vi "S2DS_User Instrument Initialize VIs.vi"(3 "error in":errorcluster, 4 "Port list (in)":T1, 5 "Instrument Info (in)":T2) -> (0 "error out":errorcluster, 1 "Port lists (out)":T1, 2 "Instrument info (out)":T2)   [LabVIEW 2025]
uses:
  TYPE DEFS/S2DS_Instrument Info.ctl
  TYPE DEFS/S2DS_Instrument parameters.ctl
  TYPE DEFS/S2DS_Port lists.ctl
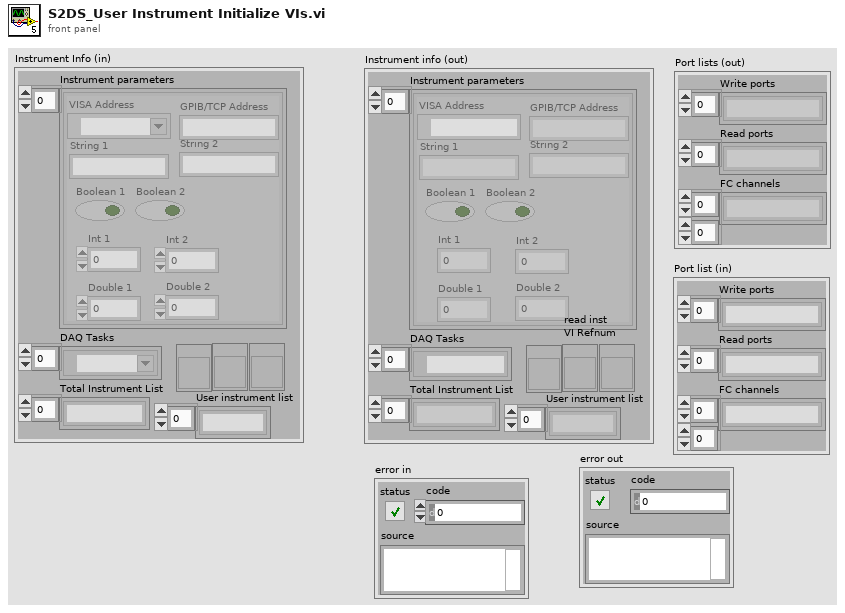
[diagram p1: front panel]
types:
  T1 = typedef "S2DS_Port lists.ctl" = cluster{"Write ports":string[], "Read ports":string[], "FC channels":string[][]}
  T2 = typedef "S2DS_Instrument Info.ctl" = cluster{"Instrument parameters":T3[], "DAQ Tasks":refnum<k21>[], "Total Instrument List":string[], "read inst \nVI Refnum":refnum<vi>, "type specifier Edit instruments VI Refnum":refnum<vi>, "type specifier write instrument VI Refnum (for type only)":refnum<vi>, "User instrument list":string[]}
  T3 = typedef "S2DS_Instrument parameters.ctl" = cluster{"VISA Address":refnum<visa-resource-name>, "GPIB/TCP Address":string, "String 1":string, "String 2":string, "Boolean 1":bool, "Boolean 2":bool, "Int 1":i32, "Int 2":i32, "Double 1":dbl, "Double 2":dbl}
  T4 = typedef "Port lists.ctl" = cluster{"Write ports":string[], "Read ports":string[], "FC channels":string[][]}
  T5 = typedef "Instrument Info.ctl" = cluster{"Instrument parameters":T6[], "DAQ Tasks":refnum<k21>[], "Instrument List":string[], "read inst \nVI Refnum":refnum<vi>, "type specifier Edit instruments VI Refnum":refnum<vi>, "type specifier write instrument VI Refnum (for type only)":refnum<vi>, "Available instrument list":string[]}
  T6 = typedef "Instrument parameters.ctl" = cluster{"VISA Address":refnum<visa-resource-name>, "GPIB/TCP Address":string, "String 1":string, "String 2":string, "Boolean 1":bool, "Boolean 2":bool, "Int 1":i32, "Int 2":i32, "Double 1":dbl, "Double 2":dbl}
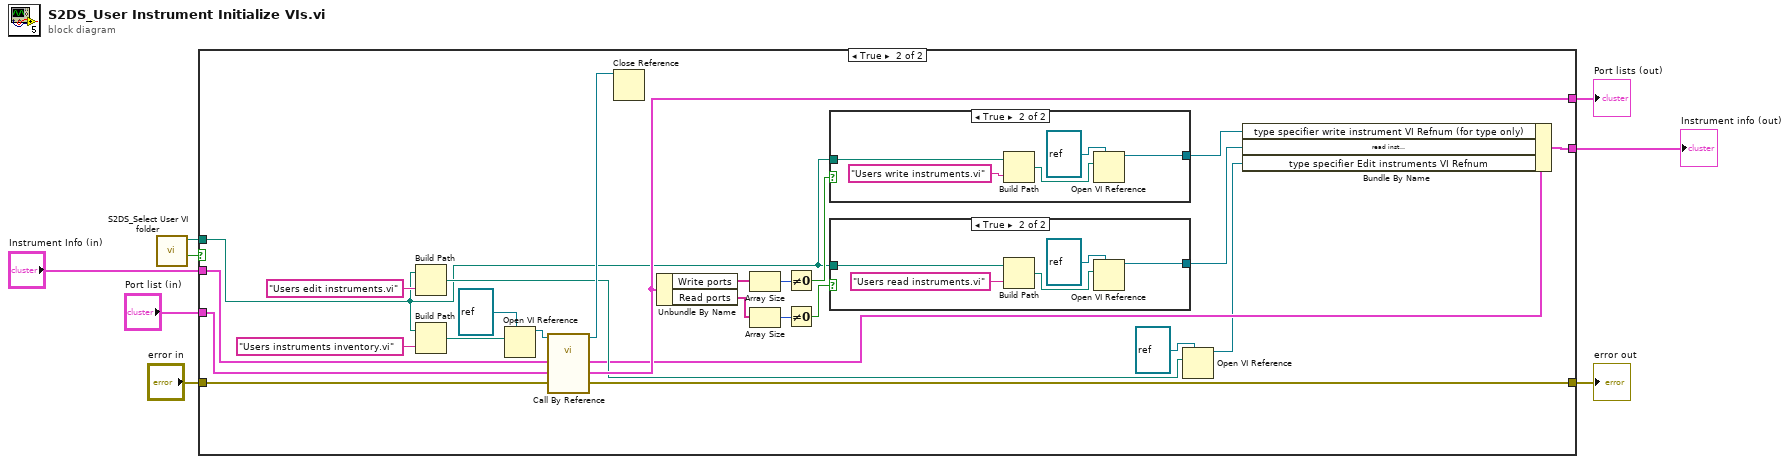
[diagram p0: block diagram]
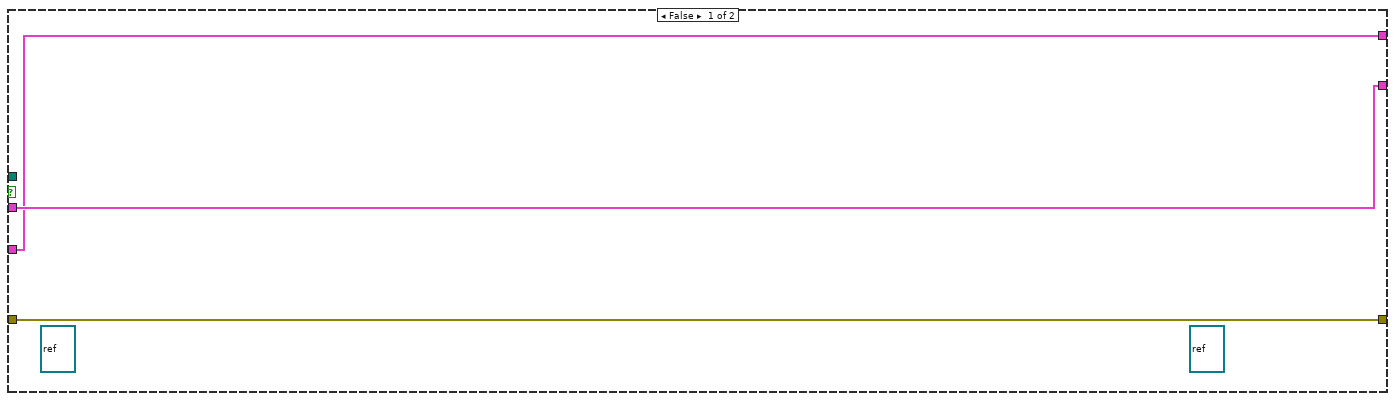
[diagram p2: hidden frame]
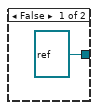
[diagram p3: hidden frame]
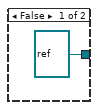
[diagram p4: hidden frame]
diagram:
  n1 = call "S2DS_Select User VI folder.vi"() -> ("Folder selected?"=w3:bool, "Path out"=w4:path)  [unwired: 10 in]
  n2 = case shown="True" w3 {
    tunnel: "Instrument Info (in)" -> [w11 w26]
    tunnel: "Port list (in)" -> [w10 w25]
    tunnel: [w11 w12] -> w6
    tunnel: [w10 w23] -> w5
    tunnel: w4 -> [_ w17]
    tunnel: "error in" -> [w9 w24]
    tunnel: [w9 w22] -> w1
    frame False {
      (unwired) refnum<vi> refnum ("type specifier VI Refnum (for type only)")
      (unwired) refnum<vi> refnum ("type specifier VI Refnum (for type only)")
    }
    frame True {
      n3 = Build Path(base path=w17, name or relative path="Users edit instruments.vi") -> (appended path=w19:path)
      n4 = Build Path(base path=w17, name or relative path="Users instruments inventory.vi") -> (appended path=w35:path)
      n5 = Open VI Reference(type specifier VI Refnum (for type only)=refnum<vi> refnum, vi path=w35) -> (vi reference=w27:refnum<vi>)  [unwired: 4 in, 1 out]
      n6 = call-by-ref "?"(reference=w27, "error in"=w24, "Port list (in)"=w25, "Instrument Info (in)"=w26) -> (reference out=w21:refnum<vi>, "Error status:"=w22:errorcluster, "Port lists (out)"=w23:T4, "Instrument info (out)"=w16:T5)  [unwired: 1 in, 1 out]
      n7 = Close Reference(reference=w21) -> ()  [unwired: 1 in, 1 out]
      n8 = Unbundle By Name(w23) -> ("Write ports"=w34:string[], "Read ports"=w30:string[])
      n9 = Array Size(array=w34) -> (size(s)=w33:i32)
      n10 = Array Size(array=w30) -> (size(s)=w31:i32)
      n11 = Not Equal To 0?(x=w33) -> (x != 0?=w32:bool)
      n12 = Not Equal To 0?(x=w31) -> (x != 0?=w29:bool)
      n13 = case shown="True" w32 {
        tunnel: w17 -> [_ w48]
        tunnel: [refnum<vi> refnum ("type specifier VI Refnum (for type only)") w44] -> w14
        frame False {
        }
        frame True {
          n14 = Build Path(base path=w48, name or relative path="Users write instruments.vi") -> (appended path=w46:path)
          n15 = Open VI Reference(type specifier VI Refnum (for type only)=refnum<vi> refnum, vi path=w46) -> (vi reference=w44:refnum<vi>)  [unwired: 4 in, 1 out]
        }
      }
      n16 = case shown="True" w29 {
        tunnel: w17 -> [_ w42]
        tunnel: [refnum<vi> refnum ("type specifier VI Refnum (for type only)") w38] -> w15
        frame False {
        }
        frame True {
          n17 = Build Path(base path=w42, name or relative path="Users read instruments.vi") -> (appended path=w40:path)
          n18 = Open VI Reference(type specifier VI Refnum (for type only)=refnum<vi> refnum, vi path=w40) -> (vi reference=w38:refnum<vi>)  [unwired: 4 in, 1 out]
        }
      }
      n19 = Open VI Reference(type specifier VI Refnum (for type only)=refnum<vi> refnum, vi path=w19) -> (vi reference=w13:refnum<vi>)  [unwired: 4 in, 1 out]
      n20 = Bundle By Name(cluster=w16, "type specifier write instrument VI Refnum (for type only)"=w14, "read inst \nVI Refnum"=w15, "type specifier Edit instruments VI Refnum"=w13) -> (w12:T5)
    }
  }
  "Instrument info (out)" <- w6
  "Port lists (out)" <- w5
  "error out" <- w1
